vi "FindSIMCOMETH.vi"(8 "error in (no error)":errorcluster caption="错误输入（无错误）") -> (0 "error out":errorcluster caption="错误输出", 3 "Result":bool)   [LabVIEW 2013]
panel:
  out "standard output":string caption="标准输出"
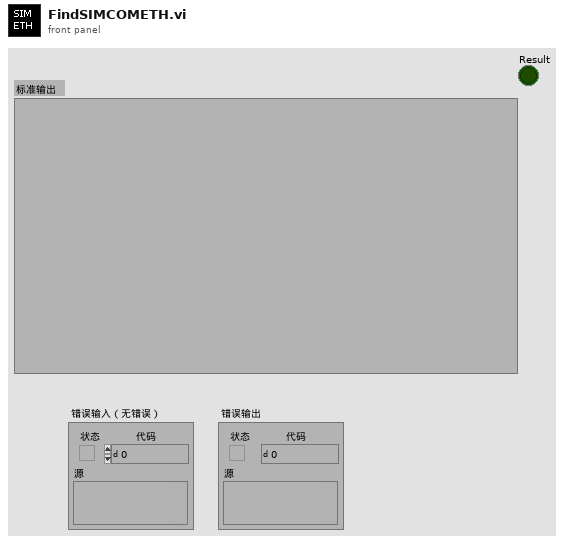
[diagram p1: front panel]
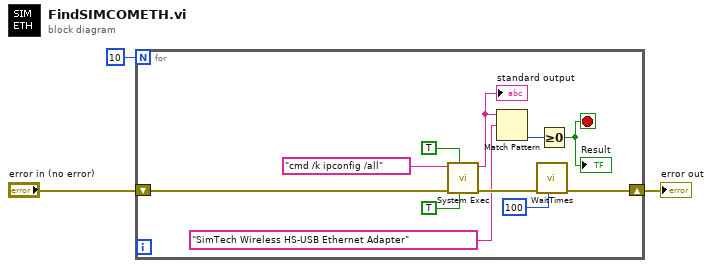
[diagram p0: block diagram]
diagram:
  n1 = for {
    N: 10 -> [_]
    shift-right: [w9] -> w1
    shift-left: "error in (no error)" -> [w12]
    stop <- w4 stop-if-true
    n2 = call <vilib>:"System Exec.vi"("run minimized? (F)"=TRUE, "wait until completion? (T)"=TRUE, "error in (no error)"=w12, "command line"="cmd /k ipconfig /all") -> ("error out"=w10:errorcluster, "standard output"=w7:string)  [unwired: 4 in, 2 out]
    "standard output" <- w7
    n3 = Match Pattern(string=w7, regular expression="SimTech Wireless HS-USB Ethernet Adapter" ("正则表达式")) -> (offset past match=w5:i32)  [unwired: 1 in, 3 out]
    n4 = call "WaitTimes.vi"("WaitTimes"=u32 100, "error in (no error)"=w10) -> ("error out"=w9:errorcluster)  [unwired: 9 in]
    n5 = Greater Or Equal To 0?(x=w5) -> (x >= 0?=w4:bool)
    "Result" <- w4
  }
  "error out" <- w1
